vi "CheckSizes.vi"(3 "Constant":u8, 4 "Image 2":T1 {"Dialogs" format="%.0b"}, 5 "Image":T1 {"Dialogs" format="%.0b"}) -> (0 "Image template":T1 {"Dialogs" format="%.0b"}, 1 "Image 2 data":u8[](array[numeric]), 2 "Image 1 data":i32[](array[numeric]))   [LabVIEW 2024]
uses:
  <userlib>/ImageProcessing/QTLIB_2595_LV86/QT_Image.ctl
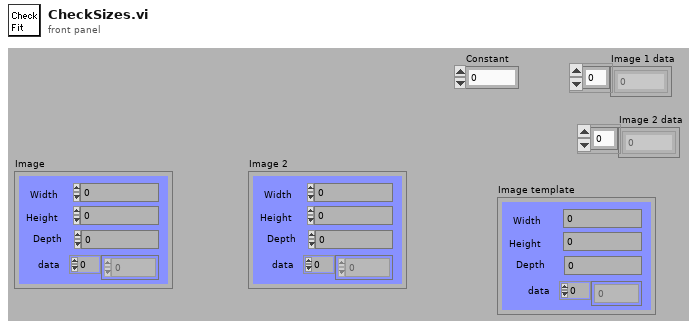
[diagram p1: front panel]
types:
  T1 = typedef "QT_Image.ctl" = cluster{"Width":i32, "Height":i32, "Depth":i32, "data":u8[], "Compressed data":u8[], "Color table":u32[], "Duration":i32, "Options":i32, "Timestamp":i32, "ID":i32, "Reserved":i32, "Dialogs":u32}
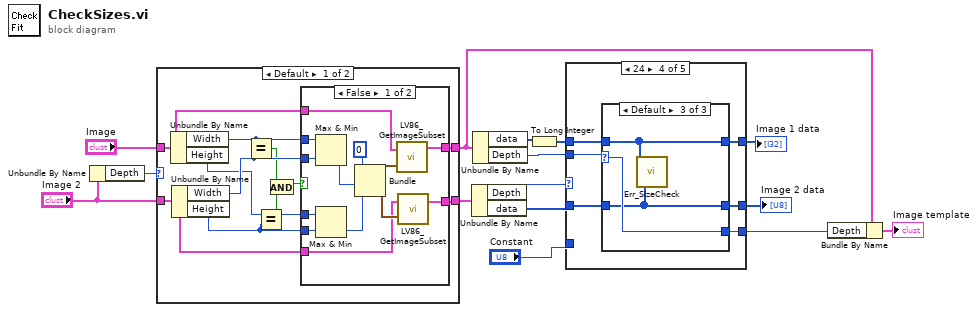
[diagram p0: block diagram]
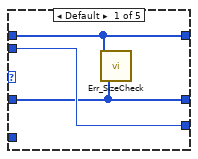
[diagram p4: hidden frame]
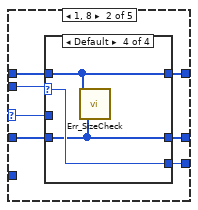
[diagram p5: hidden frame]
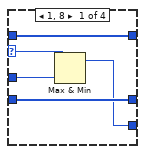
[diagram p6: hidden frame]
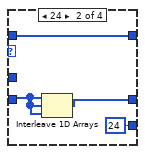
[diagram p7: hidden frame]
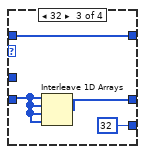
[diagram p8: hidden frame]
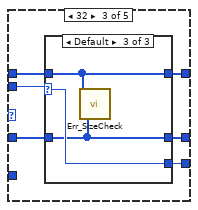
[diagram p9: hidden frame]
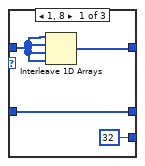
[diagram p10: hidden frame]
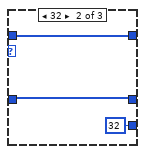
[diagram p11: hidden frame]
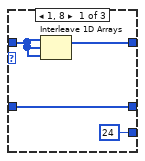
[diagram p12: hidden frame]
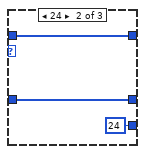
[diagram p13: hidden frame]
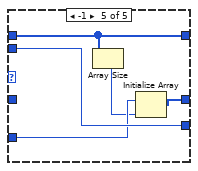
[diagram p14: hidden frame]
diagram:
  n1 = Unbundle By Name("Image 2") -> ("Depth"=w7:i32)
  n2 = case shown="Default" w7 {
    tunnel: [w24 w42] -> w6
    tunnel: "Image 2" -> [w23 w42]
    tunnel: [w25 w41] -> w3
    tunnel: "Image" -> [w26 w41]
    frame Default {
      n3 = Unbundle By Name(w26) -> ("Width"=w22:i32, "Height"=w20:i32)
      n4 = Unbundle By Name(w23) -> ("Width"=w21:i32, "Height"=w19:i32)
      n5 = Equal?(x=w22, y=w21) -> (x = y?=w17:bool)
      n6 = Equal?(x=w20, y=w19) -> (x = y?=w18:bool)
      n7 = And(x=w17, y=w18) -> (x .and. y?=w16:bool)
      n8 = case shown="False" w16 {
        tunnel: w26 -> [w38 w40]
        tunnel: [w34 w40] -> w25
        tunnel: [w33 w39] -> w24
        tunnel: w23 -> [w31 w39]
        tunnel: w22 -> [w30 _]
        tunnel: w21 -> [w29 _]
        tunnel: w20 -> [w28 _]
        tunnel: w19 -> [w27 _]
        frame False {
          w35 = 0
          n9 = Max & Min(x=w30, y=w29) -> (min(x,y)=w36:i32)  [unwired: 1 out]
          n10 = Max & Min(x=w28, y=w27) -> (min(x,y)=w37:i32)  [unwired: 1 out]
          n11 = Bundle(w35, w35, w36, w37) -> (w32:cluster{i32, i32, i32, i32})  [unwired: 1 in]
          n12 = call <userlib>:"LV86_GetImageSubset.vi"("ROI"=w32, "Image In"=w38) -> ("Image out"=w34:T1)  [unwired: 1 in]
          n13 = call <userlib>:"LV86_GetImageSubset.vi"("ROI"=w32, "Image In"=w31) -> ("Image out"=w33:T1)  [unwired: 1 in]
        }
        frame True {
        }
      }
    }
    frame -1 {
      # "constant"
    }
  }
  n14 = Unbundle By Name(w6) -> ("Depth"=w9:i32, "data"=w8:u8[])
  n15 = Unbundle By Name(w3) -> ("data"=w10:u8[], "Depth"=w12:i32)
  n16 = To Long Integer(number=w10) -> (32bit integer=w11:i32[])
  n17 = case shown="24" w9 {
    selector: w9 -> [_ w46 _ _ _]
    tunnel: w11 -> [w44 w52 w74 w90 w102]
    tunnel: "Constant" -> [_ _ _ _ w104]
    tunnel: w8 -> [w43 w51 w73 w89 _]
    tunnel: w12 -> [w45 w50 w72 w88 w105]
    tunnel: [w45 w49 w71 w87 w105] -> w2
    tunnel: [w44 w48 w70 w86 w102] -> w13
    tunnel: [w43 w47 w69 w85 w103] -> w14
    frame Default {
      n18 = call <userlib>:"Err_SizeCheck.vi"("data 2"=w43, "data"=w44) -> ()  [unwired: 2 out]
    }
    frame 1, 8 {
      n19 = case shown="Default" w50 {
        selector: w50 -> [w55 _ _ w68]
        tunnel: w52 -> [w57 w58 w62 w67]
        tunnel: w51 -> [w56 w61 w64 w66]
        tunnel: [w53 u8 24 u8 32 w68] -> w49
        tunnel: [w57 w58 w62 w67] -> w48
        tunnel: [w56 w59 w63 w66] -> w47
        tunnel: w46 -> [w54 _ _ _]
        frame 1, 8 {
          n20 = Max & Min(x=w55, y=w54) -> (max(x,y)=w53:i32)  [unwired: 1 out]
        }
        frame 24 {
          n21 = Interleave 1D Arrays(w61, w61, w61) -> (w59:u8[])
        }
        frame 32 {
          n22 = Interleave 1D Arrays(w64, w64, w64, w64) -> (w63:u8[])
        }
        frame Default {
          n23 = call <userlib>:"Err_SizeCheck.vi"("data 2"=w66, "data"=w67) -> ()  [unwired: 2 out]
        }
      }
    }
    frame 32 {
      n24 = case shown="Default" w72 {
        selector: w72 -> [_ _ w84]
        tunnel: w74 -> [w77 w80 w83]
        tunnel: w73 -> [w75 w79 w82]
        tunnel: [32 ("Depth") u8 32 w84] -> w71
        tunnel: [w76 w80 w83] -> w70
        tunnel: [w75 w79 w82] -> w69
        frame 1, 8 {
          n25 = Interleave 1D Arrays(w77, w77, w77, w77) -> (w76:i32[])
        }
        frame 32 {
        }
        frame Default {
          n26 = call <userlib>:"Err_SizeCheck.vi"("data 2"=w82, "data"=w83) -> ()  [unwired: 2 out]
        }
      }
    }
    frame 24 {
      n27 = case shown="Default" w88 {
        selector: w88 -> [_ _ w100]
        tunnel: w90 -> [w93 w96 w99]
        tunnel: w89 -> [w91 w95 w98]
        tunnel: [24 ("Depth") u8 24 w100] -> w87
        tunnel: [w92 w96 w99] -> w86
        tunnel: [w91 w95 w98] -> w85
        frame 1, 8 {
          n28 = Interleave 1D Arrays(w93, w93, w93) -> (w92:i32[])
        }
        frame 24 {
        }
        frame Default {
          n29 = call <userlib>:"Err_SizeCheck.vi"("data 2"=w98, "data"=w99) -> ()  [unwired: 2 out]
        }
      }
    }
    frame -1 {
      n30 = Array Size(array=w102) -> (size(s)=w101:i32)
      n31 = Initialize Array(w104, w101) -> (w103:u8[])
    }
  }
  "Image 2 data" <- w14
  "Image 1 data" <- w13
  n32 = Bundle By Name(cluster=w3, "Depth"=w2) -> (→"Image template":T1)
